vi "Hipot_ReadResult.vi"(8 "Error In":errorcluster, 10 "PORT":string, 11 "Limit":string="Pass") -> (0 "Error Out":errorcluster, 2 "Result":bool, 3 "Data":string)   [LabVIEW 2013]
uses:
  MainProgram/Control/Buffer.vi
panel:
  out "read buffer":string
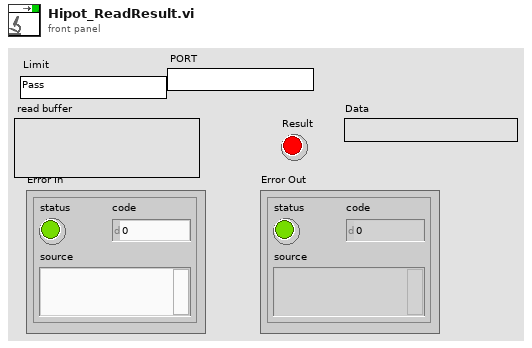
[diagram p1: front panel]
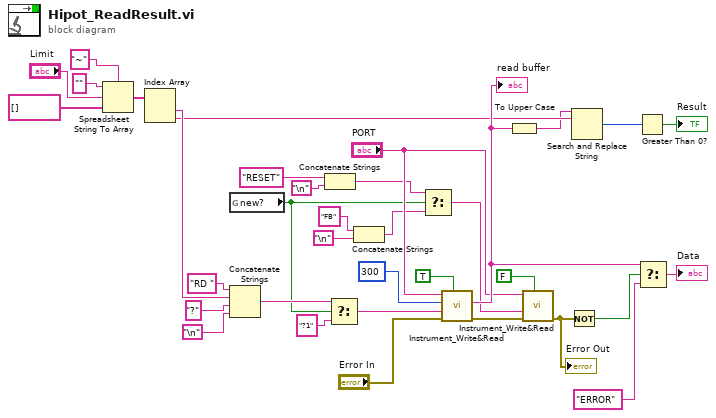
[diagram p0: block diagram]
diagram:
  n1 = Spreadsheet String To Array(delimiter (Tab)="~", format string="", spreadsheet string="Limit", array type (2D Dbl)=string[] []) -> (array=w24:string[])
  n2 = Index Array(array=w24) -> (element #1=w23:string, element #2=w21:string)  [unwired: 2 in]
  n3 = global read "Buffer.vi" "new?"() -> (w1:bool)
  n4 = Concatenate Strings("RD " ("写入缓冲区"), w23, "?" ("写入缓冲区"), "\n") -> (w13:string)
  n5 = Concatenate Strings("RESET" ("写入缓冲区"), "\n") -> (w10:string)
  n6 = Select(t=w13, s=w1, f="?1") -> (s? t:f=w12:string)
  n7 = Concatenate Strings("FB" ("Characters to Write"), "\n") -> (w3:string)
  n8 = Select(t=w10, s=w1, f=w3) -> (s? t:f=w6:string)
  n9 = call "Instrument_Write&Read.vi"("Read?"=TRUE, "Error In"="Error In", "CMD"=w12, "wait ms"=300, "PORT"="PORT") -> ("Error Out"=w31:errorcluster, "read buffer"=w30:string)  [unwired: 5 in]
  "read buffer" <- w30
  n10 = To Upper Case(1:w30) -> (0:w17:string)
  n11 = call "Instrument_Write&Read.vi"("Read?"=FALSE, "Error In"=w31, "CMD"=w6, "PORT"="PORT") -> ("Error Out"=w14:errorcluster)  [unwired: 6 in, 1 out]
  "Error Out" <- w14
  n12 = Not(x=w14) -> (.not. x?=w34:bool)
  n13 = Search and Replace String(input string=w17, search string=w21) -> (number of replacements=w19:i32)  [unwired: 6 in, 3 out]
  n14 = Greater Than 0?(x=w19) -> (x > 0?=→"Result":bool)
  n15 = Select(t=w30, s=w34, f="ERROR") -> (s? t:f=→"Data":string)
